vi "Test_Draw_To_Picture_Greyscale.vi"(8 "error in (no error)":errorcluster, 11 "Test Case In":refnum<class "Image.lvclass">) -> (0 "error out":errorcluster, 3 "Test Case Out":refnum<class "Image.lvclass">)   [LabVIEW 2020, in "g_ar_toolkit.test.lvlib" / "Image.lvclass"]
uses:
  Image.lvclass
  Image.lvclass/Image.ctl
  g_ar_toolkit.image/g_ar_toolkit.image.lvlib
  g_ar_toolkit.image/Image Size (Fixed).ctl
  g_ar_toolkit.image/Image Point (Fixed).ctl
  g_ar_toolkit.image/CreateEmptyImageGreyscale.vi
  4993e8ee-a06a-463a-9684-69129f64d5ce.vi
panel:
  out "Actual":picture
  out "Expected":picture
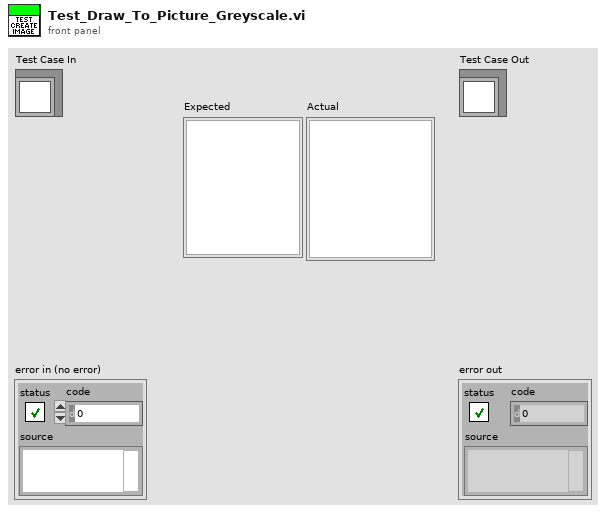
[diagram p1: front panel]
types:
  T1 = typedef "g_ar_toolkit.image.lvlib/Image Point (Fixed).ctl" = cluster{"x":i32, "y":i32}
  T2 = typedef "g_ar_toolkit.image.lvlib/Image Size (Fixed).ctl" = cluster{"Width":u16, "Height":u16}
  T3 = typedef "imagedata.ctl" = cluster{"image type":i32, "image depth":i32, "image":u8[], "mask":u8[], "colors":u32[], "Rectangle":cluster{"left":i16, "top":i16, "right":i16, "bottom":i16}}
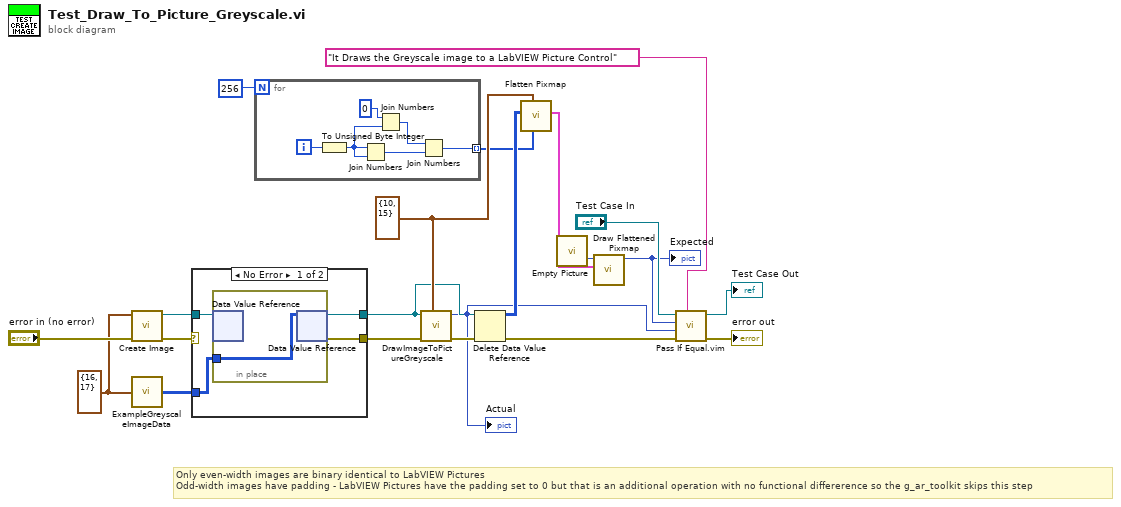
[diagram p0: block diagram]
diagram:
  w11 = T1 {"x"=10, "y"=15} ("Top-Left (0,0)")
  w3 = T2 {"Width"=16, "Height"=17} ("Preallocated Image Size (Default - 0,0)")
  # "Only even-width images are binary identical to LabVIEW Pictures\nOdd-width images have padding - LabVIEW Pictures have the padding set to 0 but that is an additional operation with no functional differerence so the g_ar_toolkit skips this step"
  n1 = call-poly "Create Image.vi"("error in (no error)"="error in (no error)", "Preallocated Image Size (Default 0,0)"=w3) -> ("error out"=w15:errorcluster, "New Greyscale Image"=w16:refnum<data-value>)  [unwired: 8 in]
  n2 = call "ExampleGreyscaleImageData.vi"("Image Size"=w3) -> ("GreyscaleImage"=w8:u8[][])
  n3 = case shown="No Error" w15 {
    selector: w15 -> [_ w27]
    tunnel: w16 -> [w25 w28]
    tunnel: [w24 w28] -> w4
    tunnel: [w23 w27] -> w13
    tunnel: w8 -> [w22 _]
    frame No Error {
      n4 = in-place {
        in-place-border: w22 -> [w26]
        n5 = in-place-dvr #1(w25) -> ()  [unwired: 2 out]
        n6 = in-place-dvr #1(w26) -> (w24:refnum<data-value>, w23:errorcluster)
      }
    }
    frame Error {
    }
  }
  n7 = for {
    N: 256 -> [_]
    tunnel: [w33] -> w5 mode=indexing
    i -> [w34]
    n8 = To Unsigned Byte Integer(number=w34) -> (unsigned 8bit integer=w30:u8)
    n9 = Join Numbers(hi=w30, lo=w30) -> ((hi.lo)=w32:u16)
    n10 = Join Numbers(hi=u8 0, lo=w30) -> ((hi.lo)=w31:u16)
    n11 = Join Numbers(hi=w31, lo=w32) -> ((hi.lo)=w33:u32)
  }
  n12 = call "DrawImageToPictureGreyscale.vi"("Image Draw Offset (Default 0,0)"=w11, "error in (no error)"=w13, "Greyscale Image Source"=w4) -> ("error out"=w12:errorcluster, "Picture"=w1:picture)  [unwired: 7 in]
  "Actual" <- w1
  n13 = Delete Data Value Reference(data value reference=w4, error in=w12) -> (data value=w7:u8[][], error out=w14:errorcluster)
  n14 = call <vilib>:"Flatten Pixmap.vi"("colors"=w5, "top left"=w11, "8-bit pixmap"=w7) -> ("image data"=w10:T3)  [unwired: 8 in]
  n15 = call "Empty Picture"() -> ("empty picture"=w9:picture)
  n16 = call <vilib>:"Draw Flattened Pixmap.vi"("image data"=w10, "picture"=w9) -> ("new picture"=w2:picture)  [unwired: 7 in]
  "Expected" <- w2
  n17 = call "Pass If Equal.vim"("Description"="It Draws the Greyscale image to a LabVIEW Picture Control", "error in (no error)"=w14, "Actual"=w1, "Expected"=w2, "LUnit Test Case In"="Test Case In") -> ("error out"=→"error out":errorcluster, "LUnit Test Case Out"=→"Test Case Out":refnum<class "Image.lvclass">)  [unwired: 5 in]
